vi "Write CH 3 Max Outputs.vi"(8 "error in (no error)":errorcluster, 10 "CH 3 Max Outputs":cluster{"Voltage (V)":dbl, "Current (A)":dbl}={"Voltage (V)"=5.0, "Current (A)"=3.0}, 11 "2230G in":refnum<class "2230G.lvclass">) -> (0 "error out":errorcluster, 3 "2230G out":refnum<class "2230G.lvclass">)   [LabVIEW 2018, in "2230G.lvlib" / "2230G.lvclass"]
uses:
  2230G.lvclass
  2230G.lvclass/2230G.ctl
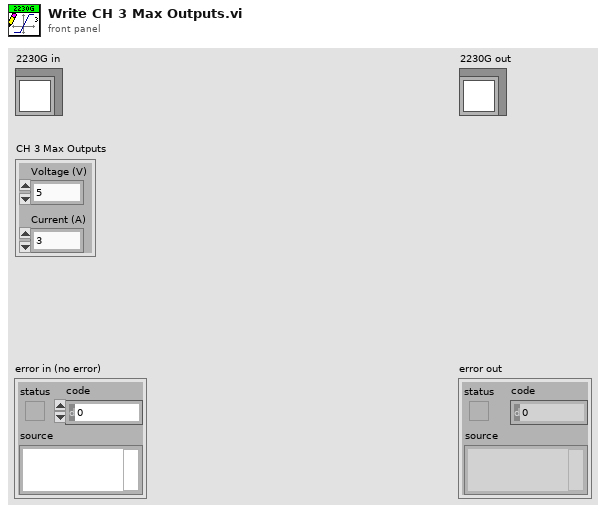
[diagram p1: front panel]
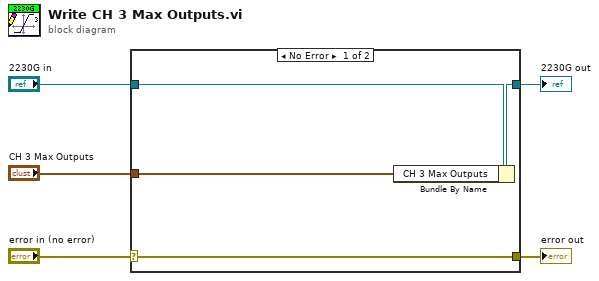
[diagram p0: block diagram]
diagram:
  n1 = case shown="No Error" "error in (no error)" {
    selector: "error in (no error)" -> [w9 w10]
    tunnel: [w9 w10] -> w4
    tunnel: [w7 w11] -> w2
    tunnel: "2230G in" -> [w8 w11]
    tunnel: "CH 3 Max Outputs" -> [w6 _]
    frame No Error {
      n2 = Bundle By Name(cluster=w8, "CH 3 Max Outputs"=w6) -> (w7:refnum<class "2230G.lvclass">)
    }
    frame Error {
    }
  }
  "error out" <- w4
  "2230G out" <- w2
